vi "PID Test X-Axis.vi"() -> ()   [LabVIEW 2017]
uses:
  <vilib>/myRIO/Common/Instrument Driver Framework/myRIO v1.0/UART/vis/myRIO v1.0 Close UART.vi
  <vilib>/addons/control/pid/pid.llb/PID Control Input Filter (DBL).vi
  <vilib>/addons/control/pid/pid.llb/PID (DBL).vi
  <vilib>/myRIO/Common/Instrument Driver Framework/Utilities/vis/FPGA Ref Manager.vi
  <vilib>/myRIO/Common/Instrument Driver Framework/myRIO v1.0/myRIO v1.0 Reset FPGA.vi
  <vilib>/myRIO/Common/Instrument Driver Framework/myRIO v1.0/IRQ/vis/myRIO v1.0 IRQ Info FGV.vi
  <vilib>/myRIO/Common/Instrument Driver Framework/myRIO v1.0/IRQ/vis/myRIO v1.0 Timer IRQ Info FGV.vi
  <vilib>/myRIO/Common/Instrument Driver Framework/myRIO v1.0/IRQ/vis/myRIO v1.0 ISR Agent.vi
  <vilib>/addons/control/pid/NI_PID_pid.lvlib
  <vilib>/myRIO/Instrument Drivers/Utilities/Utilities.lvlib
panel:
  out "Sensor Output":cluster{dbl, "output":dbl}(graph)
  out "Motion Data":T1
  out "Velocity Set Pt":dbl
  in  "FWD/RVS":bool
  out "Time (s)":dbl
  out "Output String":string
  out "PID Output":dbl(graph)
  out "SP & PV":T2(graph)
  in  "PID gains":T3={"proportional gain (Kc)"=1.0, "integral time (Ti, min)"=0.01, "derivative time (Td, min)"=0.0} {"derivative time (Td, min)" format="%.4f"; "integral time (Ti, min)" format="%.4f"; "proportional gain (Kc)" format="%.3f"}
  out "dt out (s)":dbl format="%.3f"
  in  "Frequency":dbl
  in  "Velocity Set Pt":dbl
  in  "stop":bool
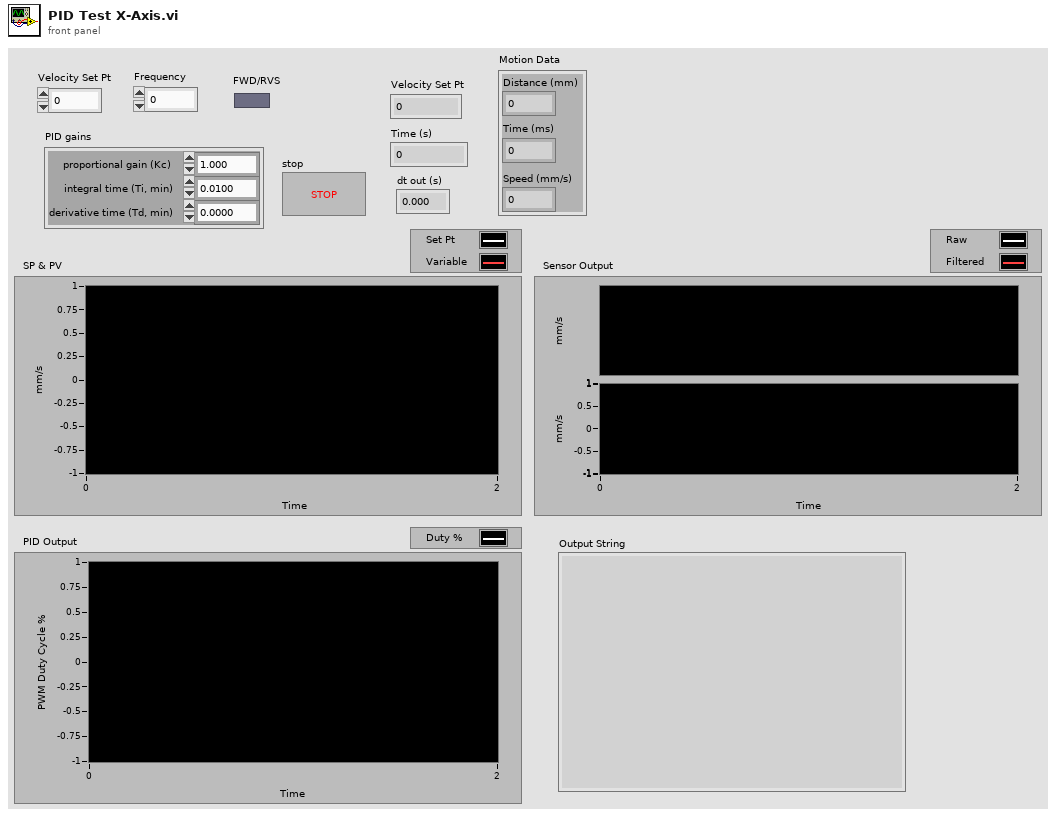
[diagram p1: front panel]
types:
  T1 = cluster{"Distance (mm)":dbl, "Time (ms)":u32, "Speed (mm/s)":dbl}
  T2 = cluster{"Velocity Set Pt":dbl, "Velocity (mm/s)":dbl}
  T3 = cluster{"proportional gain (Kc)":dbl, "integral time (Ti, min)":dbl, "derivative time (Td, min)":dbl}
  T4 = cluster{"Velocity Set Pt":dbl, "Velocity (mm/s)":dbl}[]
  T5 = typedef "Encoder Cluster.ctl" = cluster{"Y-axis rev count":dbl, "Y-axis distance":dbl, "X-axis rev count":dbl, "X-axis distance":dbl, "Y-axis direction":T6, "X-axis direction":T6, "X-counter val":i32, "Y-counter val":i32}
  T6 = typedef "Encoder Count Direction Enum.ctl" = enum16{"Counting Up", "Counting Down"}
  T7 = cluster{dbl, "Velocity Set Pt":dbl, dbl, "output":dbl, "proportional gain (Kc)":dbl, "integral time (Ti, min)":dbl, "derivative time (Td, min)":dbl}
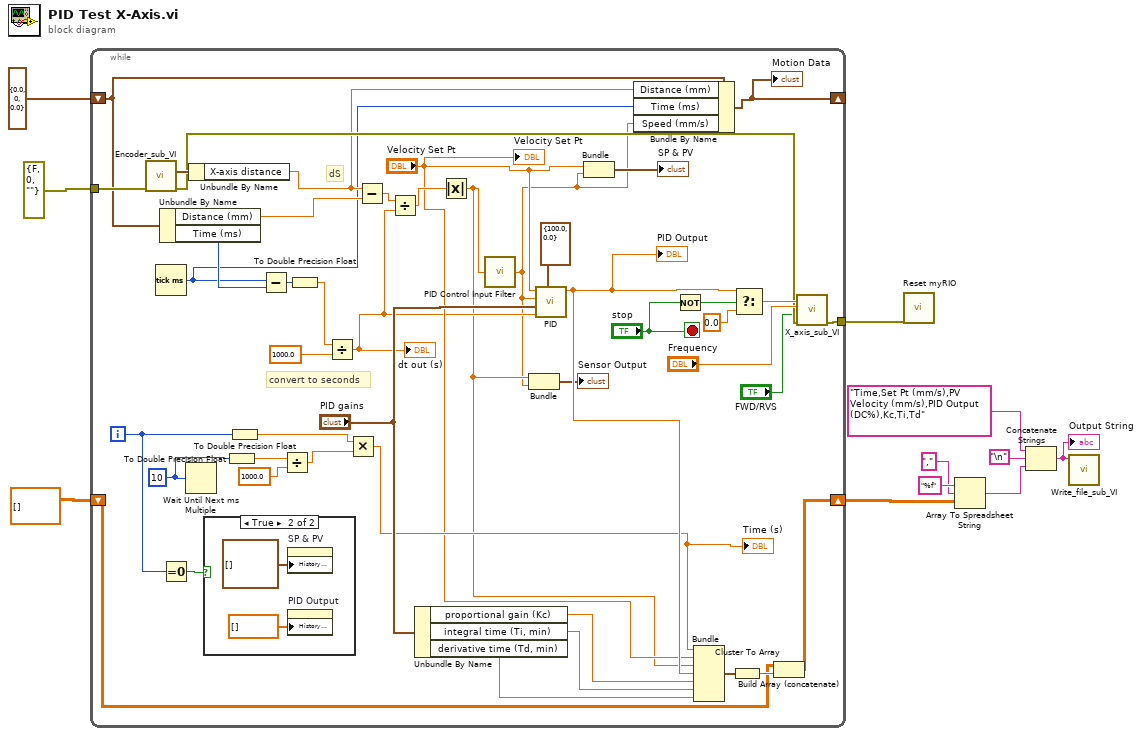
[diagram p0: block diagram]
diagram:
  n1 = while {
    shift-right: [w38] -> w4
    shift-left: dbl[][] [] ("element") -> [w39]
    tunnel: errorcluster {"status"=FALSE, "code"=0, "source"=""} ("error constant") -> [w37]
    tunnel: [w35] -> w2
    shift-right: [w16] -> _
    shift-left: T1 {"Distance (mm)"=0.0, "Time (ms)"=0, "Speed (mm/s)"=0.0} ("Motion Data") -> [w20]
    i -> [w23]
    stop <- "stop" stop-if-true
    w26 = u32 10 ("millisecond multiple")
    # "dS"
    # "convert to seconds"
    n2 = call "Encoder_sub_VI.vi"("error in (no error)"=w37) -> ("error out"=w36:errorcluster, "Encoder Output"=w55:T5)  [unwired: 9 in]
    n3 = Tick Count (ms)() -> (millisecond timer value=w17:u32)
    n4 = Unbundle By Name(w20) -> ("Distance (mm)"=w21:dbl, "Time (ms)"=w18:u32)
    n5 = Equal To 0?(x=w23) -> (x = 0?=w24:bool)
    n6 = Wait Until Next ms Multiple(millisecond multiple=w26) -> ()  [unwired: 1 out]
    n7 = Unbundle By Name(w55) -> ("X-axis distance"=w19:dbl)
    n8 = case shown="True" w24 {
      frame False {
      }
      frame True {
        n9 = property on="SP & PV" class="WFChart (strict)"("History Data"=T4 []) -> ()  [unwired: 2 in, 2 out]
        n10 = property on="PID Output" class="WFChart (strict)"("History Data"=dbl[] []) -> ()  [unwired: 2 in, 2 out]
      }
    }
    n11 = To Double Precision Float(number=w26) -> (double precision float=w34:dbl)
    n12 = To Double Precision Float(number=w23) -> (double precision float=w27:dbl)
    n13 = Subtract(x=w17, y=w18) -> (x-y=w45:u32)
    n14 = Divide(x=w34, y=1000.0) -> (x/y=w29:dbl)
    n15 = To Double Precision Float(number=w45) -> (double precision float=w44:dbl)
    n16 = Divide(x=w44, y=1000.0) -> (x/y=w15:dbl)
    "dt out (s)" <- w15
    n17 = Multiply(x=w27, y=w29) -> (x*y=w28:dbl)
    "Time (s)" <- w28
    n18 = Subtract(x=w19, y=w21) -> (x-y=w53:dbl)
    n19 = Divide(x=w53, y=w15) -> (x/y=w52:dbl)
    n20 = Unbundle By Name("PID gains") -> ("proportional gain (Kc)"=w32:dbl, "integral time (Ti, min)"=w31:dbl, "derivative time (Td, min)"=w30:dbl)
    n21 = Absolute Value(x=w52) -> (abs(x)=w13:dbl)
    n22 = call-poly <vilib>:"PID Control Input Filter.vi"("input"=w13) -> ("output"=w12:dbl)  [unwired: 4 in]
    n23 = Bundle(w13, "output"=w12) -> (→"Sensor Output":cluster{dbl, "output":dbl})  [unwired: 1 in]
    n24 = call-poly <vilib>:"PID.vi"("output range"=cluster{"output high":dbl, "output low":dbl} {"output high"=100.0, "output low"=0.0}, "dt (s)"=w15, "PID gains"="PID gains", "process variable"=w12, "setpoint"="Velocity Set Pt") -> ("output"=w43:dbl)  [unwired: 5 in, 1 out]
    "PID Output" <- w43
    n25 = Bundle("Velocity Set Pt"="Velocity Set Pt", "output"=w12) -> (→"SP & PV":cluster{"Velocity Set Pt":dbl, "output":dbl})  [unwired: 1 in]
    n26 = Bundle By Name(cluster=w20, "Distance (mm)"=w19, "Time (ms)"=w17, "Speed (mm/s)"=w12) -> (w16:T1)
    "Motion Data" <- w16
    n27 = Not(x="stop") -> (.not. x?=w50:bool)
    n28 = Bundle(w28, "Velocity Set Pt"="Velocity Set Pt", w13, "output"=w43, "proportional gain (Kc)"=w32, "integral time (Ti, min)"=w31, "derivative time (Td, min)"=w30) -> (w41:T7)  [unwired: 1 in]
    n29 = Cluster To Array(cluster=w41) -> (array=w40:dbl[])
    n30 = Select(t=w43, s=w50, f=0.0) -> (s? t:f=w48:dbl)
    n31 = Build Array (concatenate)(w39, w40) -> (w38:dbl[][])
    n32 = call "X_axis_sub_VI.vi"("error in (no error)"=w36, "FWD/RVS"="FWD/RVS", "Frequency"="Frequency", "Duty Cycle %"=w48) -> ("error out"=w35:errorcluster)  [unwired: 7 in]
    "Velocity Set Pt" <- "Velocity Set Pt"
  }
  n33 = call <vilib>:"Reset myRIO.vi"("error in (no error)"=w2) -> ()  [unwired: 10 in, 1 out]
  n34 = Array To Spreadsheet String(delimiter (Tab)=",", array=w4, 3:"%f" ("format string")) -> (spreadsheet string=w10:string)
  n35 = Concatenate Strings("Time,Set Pt (mm/s),PV Velocity (mm/s),PID Output (DC%),Kc,Ti,Td", "\n", w10) -> (w9:string)
  "Output String" <- w9
  n36 = call "Write_file_sub_VI.vi"("Output String"=w9) -> ()  [unwired: 9 in, 2 out]
